vi "Read TDMS Temp.vi"() -> ()   [LabVIEW 2020]
panel:
  out "Array":dbl[](array[numeric])
  out "Res Data":dbl[][](graph)
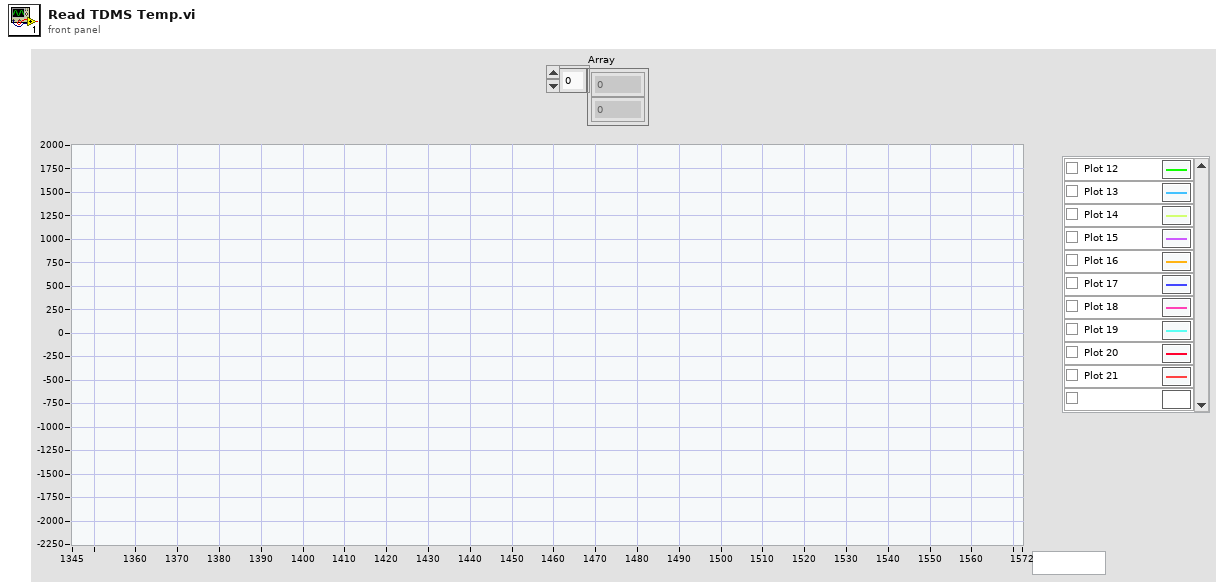
[diagram p1: front panel]
types:
  T1 = enum16{"open", "open or create", "create or replace", "create", "open (read-only)"}
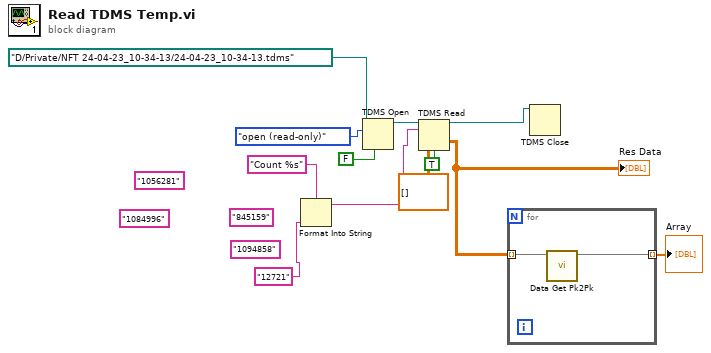
[diagram p0: block diagram]
diagram:
  (unwired) "1056281" ("input 1")
  (unwired) "1084996" ("input 1")
  (unwired) "1094858" ("input 1")
  (unwired) "845159" ("input 1")
  n1 = Format Into String(format string="Count %s", "12721" ("input 1")) -> (resulting string=w6:string)  [unwired: 2 in, 1 out]
  n2 = TDMS Open(6:FALSE ("disable buffering? (T)"), 10:T1."open (read-only)" ("operation"), 11:path "D:/Private/NFT 24-04-23_10-34-13/24-04-23_10-34-13.tdms" ("file path")) -> (3:w11:refnum<k34>)  [unwired: 4 in, 1 out]
  n3 = TDMS Read(0:w11, 5:w6, 12:dbl[][] [], 13:TRUE ("return channels in file order? (F)")) -> (4:w4:refnum<k34>, 10:w1:dbl[][])  [unwired: 4 in, 4 out]
  "Res Data" <- w1
  n4 = for {
    tunnel: w1 -> [w14] mode=indexing
    tunnel: [w13] -> w3 mode=indexing
    n5 = call "Data Get Pk2Pk.vi"("Data"=w14) -> (3:w13)  [unwired: 9 in, 1 out]
  }
  "Array" <- w3
  n6 = TDMS Close(11:w4) -> ()  [unwired: 1 in, 2 out]
